vi "DAQ DO.vi"(8 "error in":errorcluster, 10 "Relay Mode":bool[](array[boolean]), 11 "Alias":string="DUT0") -> (0 "error out":errorcluster={"status"=TRUE, "code"=91, "source"="Variant To Data in DAQ DO.vi"})   [LabVIEW 2021, in "GIP Wrappers.lvlib"]
uses:
  Load INI/Controls/DAQ_Data.ctl
  <vilib>/DAQmx/write.llb/DAQmx Write (Digital 1D Bool 1Chan 1Samp).vi
  <vilib>/DAQmx/create/channels.llb/DAQmx Create Channel (DO-Digital Output).vi
  <vilib>/DAQmx/miscellaneous.llb/DAQmx Fill In Error Info.vi
  GIP Wrappers.lvlib
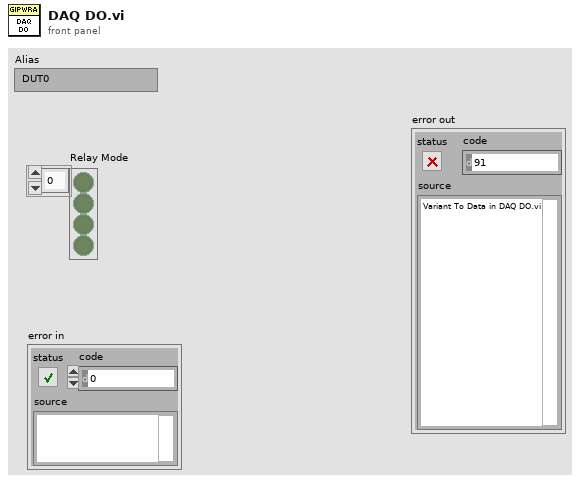
[diagram p1: front panel]
types:
  T1 = typedef "DAQ_Data.ctl" = cluster{"Alias":string, "MUX":string, "Route":string, "Channel":string}
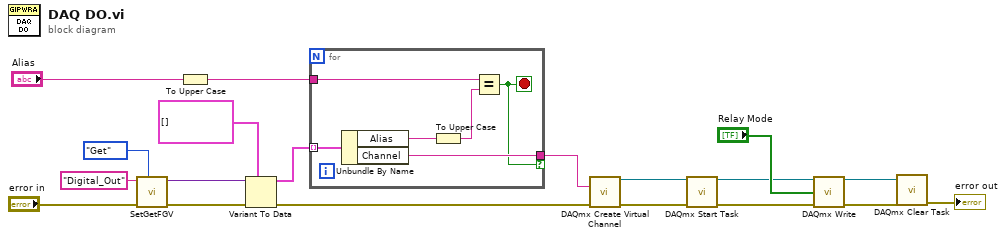
[diagram p0: block diagram]
diagram:
  n1 = call "SetGetFGV.vi"("Method (Get)"=enum16{"Get", "Set"}."Get", "error in"="error in", "FGVname"="Digital_Out" ("Name")) -> ("error out"=w15:errorcluster, "Data out"=w16:variant)  [unwired: 7 in]
  n2 = To Upper Case(1:"Alias") -> (0:w11:string)
  n3 = Variant To Data(error in=w15, type=T1[] [], Variant=w16) -> (data=w12:T1[], error out=w13:errorcluster)
  n4 = for {
    tunnel: w12 -> [w25] mode=indexing
    tunnel: [w24] -> w1 if=w21
    tunnel: w11 -> [w23]
    stop <- w21 stop-if-true
    n5 = Unbundle By Name(w25) -> ("Alias"=w22:string, "Channel"=w24:string)
    n6 = To Upper Case(1:w22) -> (0:w20:string)
    n7 = Equal?(x=w23, y=w20) -> (x = y?=w21:bool)
  }
  n8 = call-poly <vilib>:"DAQmx Create Virtual Channel.vi"("lines"=w1, "error in"=w13) -> ("task out"=w6:refnum<k21>, "error out"=w7:errorcluster)  [unwired: 12 in]
  n9 = call <vilib>:"DAQmx Start Task.vi"("task/channels in"=w6, "error in"=w7) -> ("task out"=w4:refnum<k21>, "error out"=w5:errorcluster)  [unwired: 12 in]
  n10 = call-poly <vilib>:"DAQmx Write.vi"("task/channels in"=w4, "data"="Relay Mode", "error in"=w5) -> ("task out"=w2:refnum<k21>, "error out"=w3:errorcluster)  [unwired: 10 in, 1 out]
  n11 = call <vilib>:"DAQmx Clear Task.vi"("task in"=w2, "error in"=w3) -> ("error out"=→"error out":errorcluster)  [unwired: 13 in]
